vi "FTW-Container-Support-XML-ContainerType.vi"(0 "Element Node":refnum<k20>, 11 "error in":errorcluster) -> (4 "Element Node out":refnum<k20>, 6 "Parent XPath Query":string, 8 "Parent Type":T1, 10 "XML Structure":string, 15 "error out":errorcluster)   [LabVIEW 2013, in "FTW-Container.lvclass"]
uses:
  FTW-Container.lvclass
  JSON/FTW-JSON-CompositeType.ctl
  Error/FTW-ERR-ThrowError.vi
  <resource>/objmgr/DOMUserDefRef.rc
panel:
  # "Inputs"
  # "Outputs"
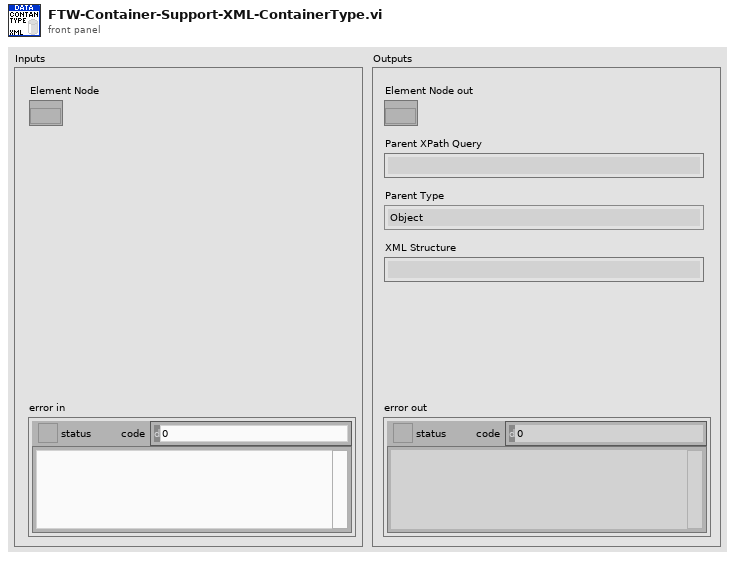
[diagram p1: front panel]
types:
  T1 = typedef "FTW-JSON-CompositeType.ctl" = enum16{"Object", "Array"}
  T2 = typedef "FTW-JSON-Datatype.ctl" = enum16{"Object", "Array", "String", "Number", "Boolean", "NULL", "<Refnum>", "<Enum>", "<Unknown>"}
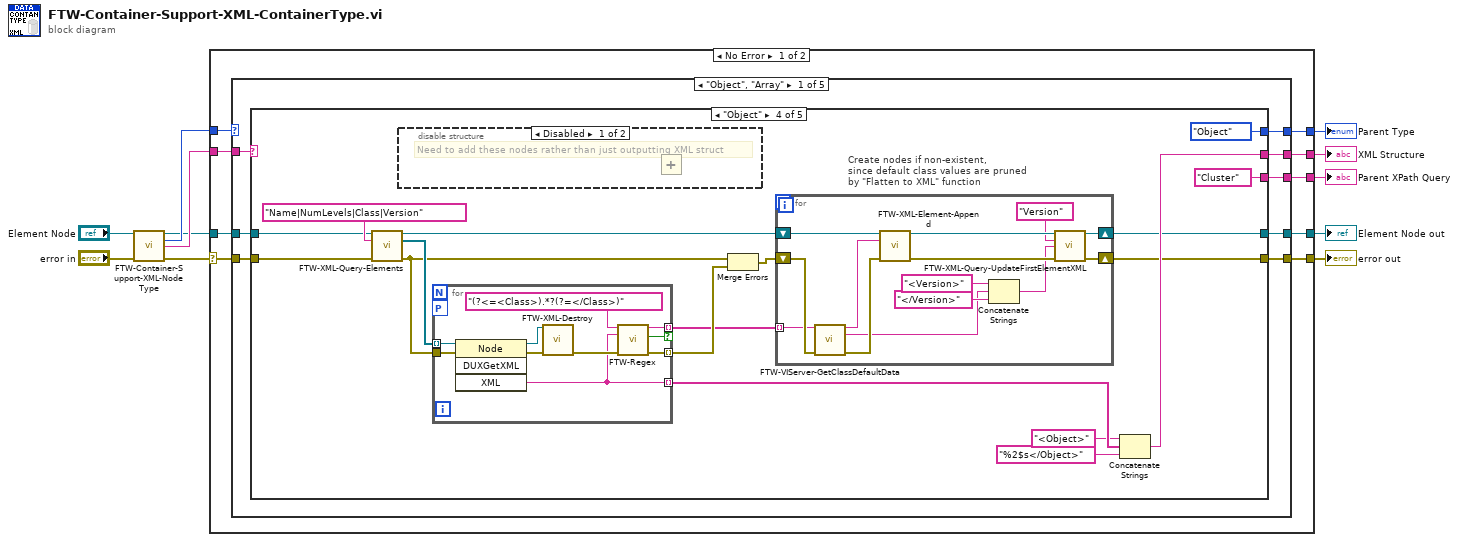
[diagram p0: block diagram]
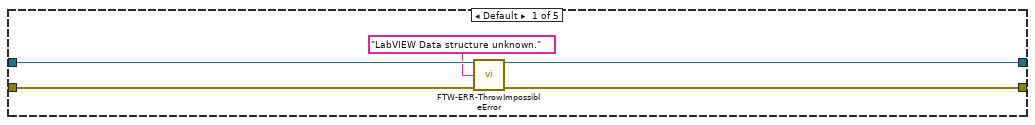
[diagram p2: hidden frame]
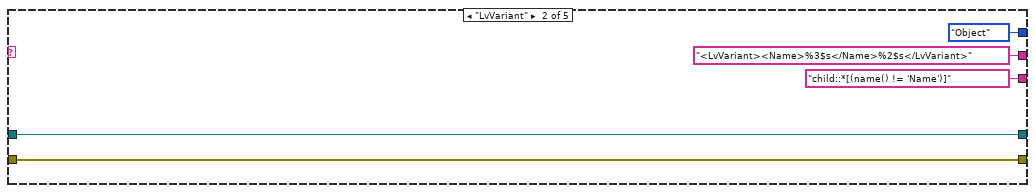
[diagram p3: hidden frame]
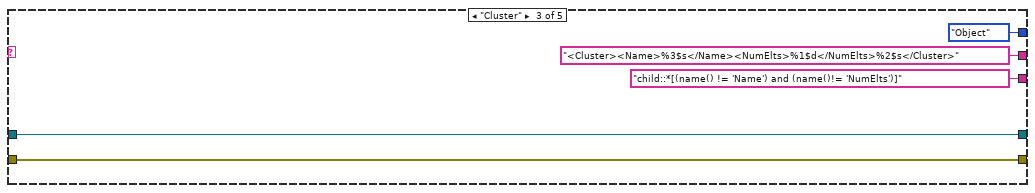
[diagram p4: hidden frame]
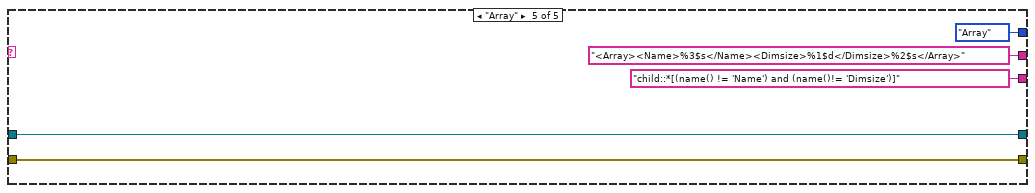
[diagram p6: hidden frame]
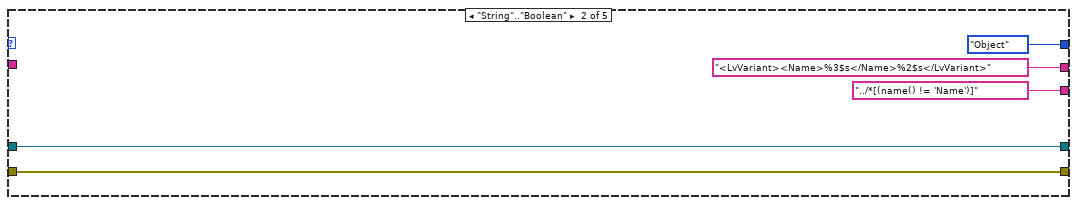
[diagram p7: hidden frame]
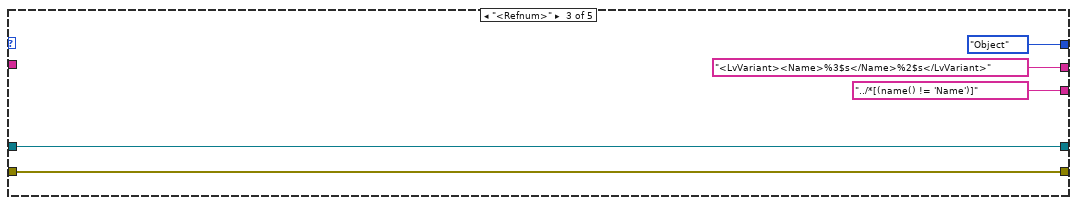
[diagram p8: hidden frame]
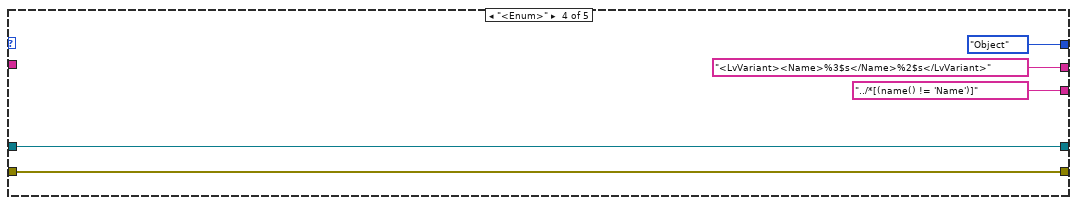
[diagram p9: hidden frame]
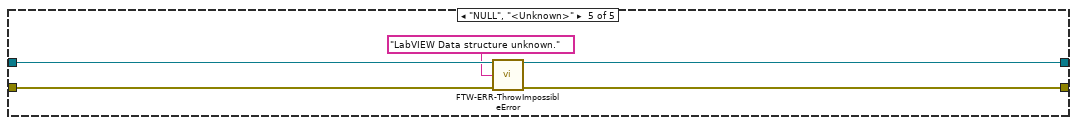
[diagram p10: hidden frame]
diagram:
  n1 = call "FTW-Container-Support-XML-NodeType.vi"("Element Node"="Element Node", "error in"="error in") -> ("Element Node out"=w2:refnum<k20>, "JSON Type"=w10:T2, "Node XML Type"=w11:string, "error out"=w1:errorcluster)  [unwired: 10 in]
  n2 = case shown="No Error" w1 {
    selector: w1 -> [w12 w108]
    tunnel: w11 -> [w20 _]
    tunnel: w10 -> [w19 _]
    tunnel: [w18 _] -> w7
    tunnel: [w17 _] -> w6
    tunnel: [w16 _] -> w5
    tunnel: [w15 w108] -> w4
    tunnel: [w14 w109] -> w3
    tunnel: w2 -> [w13 w109]
    frame No Error {
      n3 = case shown="\"Object\", \"Array\"" w19 {
        tunnel: w20 -> [w28 _ _ _ _]
        tunnel: [w27 "<LvVariant><Name>%3$s</Name>%2$s</LvVariant>" "<LvVariant><Name>%3$s</Name>%2$s</LvVariant>" "<LvVariant><Name>%3$s</Name>%2$s</LvVariant>" _] -> w17
        tunnel: [w26 "../*[(name() != 'Name')]" "../*[(name() != 'Name')]" "../*[(name() != 'Name')]" _] -> w16
        tunnel: [w25 FTW-JSON-CompositeType."Object" ("Parent Container") FTW-JSON-CompositeType."Object" ("Parent Container") FTW-JSON-CompositeType."Object" ("Parent Container") _] -> w18
        tunnel: [w24 w89 w94 w99 w104] -> w15
        tunnel: w12 -> [w23 w89 w94 w99 w105]
        tunnel: [w22 w90 w95 w100 w107] -> w14
        tunnel: w13 -> [w21 w90 w95 w100 w107]
        frame "Object", "Array" {
          n4 = case shown="\"Object\"" w28 {
            tunnel: [_ "<LvVariant><Name>%3$s</Name>%2$s</LvVariant>" "<Cluster><Name>%3$s</Name><NumElts>%1$d</NumElts>%2$s</Cluster>" w49 "<Array><Name>%3$s</Name><Dimsize>%1$d</Dimsize>%2$s</Array>"] -> w27
            tunnel: [_ "child::*[(name() != 'Name')]" "child::*[(name() != 'Name') and (name()!= 'NumElts')]" "Cluster" "child::*[(name() != 'Name') and (name()!= 'Dimsize')]"] -> w26
            tunnel: [_ FTW-JSON-CompositeType."Object" ("Parent Container") FTW-JSON-CompositeType."Object" ("Parent Container") FTW-JSON-CompositeType."Object" ("Parent Container") FTW-JSON-CompositeType."Array" ("Parent Container")] -> w25
            tunnel: [w29 w33 w38 w48 w84] -> w24
            tunnel: w23 -> [w30 w33 w38 w57 w84]
            tunnel: [w32 w34 w39 w44 w85] -> w22
            tunnel: w21 -> [w32 w34 w39 w45 w85]
            frame Default {
              n5 = call "FTW-ERR-ThrowImpossibleError.vi"("Reason this error should never happen"="LabVIEW Data structure unknown.", "error in"=w30) -> ("error out"=w29:errorcluster)  [unwired: 13 in]
            }
            frame "LvVariant" {
            }
            frame "Cluster" {
            }
            frame "Object" {
              n6 = call "FTW-XML-Query-Elements.vi"("XML Node"=w45, "XPath Query"="Name|NumLevels|Class|Version", "error in"=w57) -> ("XML Node out"=w46:refnum<k20>, "Matching Nodes"=w55:refnum<k20>[], "error out"=w54:errorcluster)  [unwired: 9 in, 1 out]
              n7 = disable-structure shown="Disabled" {
                frame Disabled {
                  # "Need to add these nodes rather than just outputting XML struct"
                  n8 = Add() -> ()  [unwired: 2 in, 1 out]
                }
                frame Enabled {
                }
              }
              n9 = for {
                tunnel: w55 -> [w81] mode=indexing
                tunnel: w54 -> [w80]
                workers-P: _ -> [_]
                tunnel: [w78] -> w53 mode=indexing
                tunnel: [w77] -> w52 mode=indexing
                tunnel: [w76] -> w43 mode=indexing if=w75
                n10 = invoke class="Node" method="DUXGetXML"(reference=w81, error in=w80) -> (reference out=w83:refnum<k20>, error out=w82:errorcluster, "XML"=w77:string)  [unwired: 2 in, 1 out]
                n11 = call "FTW-XML-Destroy.vi"("XML Node"=w83, "error in"=w82) -> ("error out"=w79:errorcluster)  [unwired: 13 in]
                n12 = call "FTW-Regex.vi"("Regular Expression"="(?<=<Class>).*?(?=</Class>)", "Input String"=w77, "error in"=w79) -> ("Match"=w76:string, "Match Found?"=w75:bool, "error out"=w78:errorcluster)  [unwired: 8 in, 2 out]
              }
              n13 = Merge Errors(w54, w53) -> (w47:errorcluster)
              n14 = for "Create nodes if non-existent,\nsince default class values are pruned\nby \"Flatten to XML\" function" {
                tunnel: w43 -> [w69] mode=indexing
                shift-right: [w66] -> w48
                shift-left: w47 -> [w72]
                shift-right: [w65] -> w44
                shift-left: w46 -> [w73]
                n15 = call "FTW-VIServer-GetClassDefaultData.vi"("Fully-Qualified Class Name"=w69, "error in"=w72) -> ("Class Data"=w70:string, "Class Version"=w61:string, "error out"=w71:errorcluster)  [unwired: 11 in]
                n16 = call "FTW-XML-Element-Append.vi"("Parent Element"=w73, "XML Element to Append"=w70, "error in"=w71) -> ("Parent Element out"=w68:refnum<k20>, "error out"=w67:errorcluster)  [unwired: 10 in, 1 out]
                n17 = Concatenate Strings("<Version>", w61, "</Version>") -> (w60:string)
                n18 = call "FTW-XML-Query-UpdateFirstElementXML.vi"("Parent Element"=w68, "XPath Query"="Version", "New XML Element"=w60, "error in"=w67) -> ("Parent Element out"=w65:refnum<k20>, "error out"=w66:errorcluster)  [unwired: 9 in, 1 out]
              }
              n19 = Concatenate Strings("<Object>", w52, "%2$s</Object>") -> (w49:string)
            }
            frame "Array" {
            }
          }
        }
        frame "String".."Boolean" {
        }
        frame "<Refnum>" {
        }
        frame "<Enum>" {
        }
        frame "NULL", "<Unknown>" {
          n20 = call "FTW-ERR-ThrowImpossibleError.vi"("Reason this error should never happen"="LabVIEW Data structure unknown.", "error in"=w105) -> ("error out"=w104:errorcluster)  [unwired: 13 in]
        }
      }
    }
    frame Error {
    }
  }
  "error out" <- w4
  "Element Node out" <- w3
  "XML Structure" <- w6
  "Parent Type" <- w7
  "Parent XPath Query" <- w5
